vi "Write MongoDB.Collection.vi"(8 "error in (no error)":errorcluster, 10 "MongoDB.Collection":refnum<k24>, 11 "MongoDB.Collection in":refnum<class "MongoDB.Collection.lvclass">) -> (0 "error out":errorcluster, 3 "MongoDB.Collection out":refnum<class "MongoDB.Collection.lvclass">)   [LabVIEW 2014, in "MongoDB.Collection.lvclass"]
uses:
  MongoDB.Collection.lvclass
  C:/Users/Richard/Documents/GitHub/mongo-labview-driver/CSharp/bin/MongoDB.Driver.Legacy.dll
  CSharp/bin/MongoDB.Driver.Legacy.dll
  MongoDB.Collection.lvclass/MongoDB.Collection.ctl
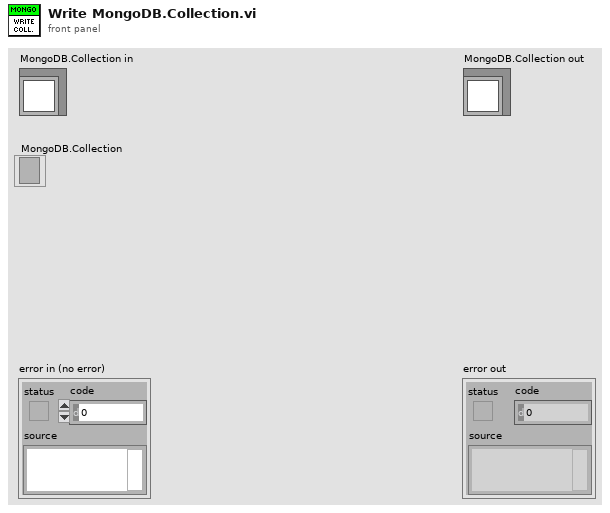
[diagram p1: front panel]
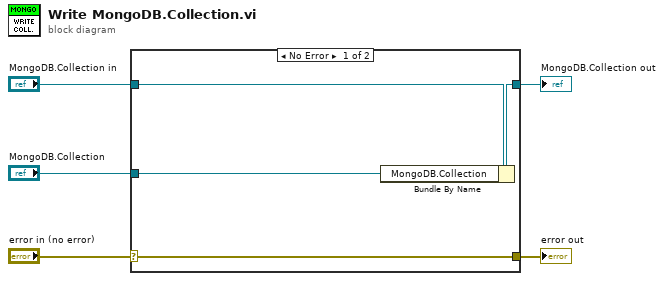
[diagram p0: block diagram]
diagram:
  n1 = case shown="No Error" "error in (no error)" {
    selector: "error in (no error)" -> [w9 w10]
    tunnel: [w9 w10] -> w4
    tunnel: [w7 w11] -> w2
    tunnel: "MongoDB.Collection in" -> [w8 w11]
    tunnel: "MongoDB.Collection" -> [w6 _]
    frame No Error {
      n2 = Bundle By Name(cluster=w8, "MongoDB.Collection"=w6) -> (w7:refnum<class "MongoDB.Collection.lvclass">)
    }
    frame Error {
    }
  }
  "error out" <- w4
  "MongoDB.Collection out" <- w2
